vi "SwapElectrodes.vi"(1 "index 2":i32=5, 2 "index 1":i32=4, 3 "Excitations in":dbl[](array[numeric])=[-7.852284145732824, -6.6524880255455034, -6.63672624222675, -6.6562009105673745, -7.978464811675144, -7.977669192926473, -7.983560531970807, -0.0001659795114891018, 0.0, 0.0, 0.0, 0.0, 0.0, 0.0, 0.0, 0.6666666666666666]) -> (0 "Excitations out":dbl[](array[numeric])=[-7.852284145732824, -6.6524880255455034, -6.63672624222675, -6.6562009105673745, -7.977669192926473, -7.978464811675144, -7.983560531970807, -0.0001659795114891018, 0.0, 0.0, 0.0, 0.0, 0.0, 0.0, 0.0, 0.6666666666666666])   [LabVIEW 2018]
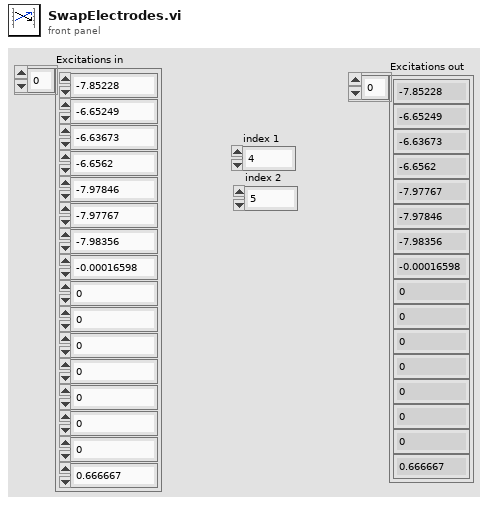
[diagram p1: front panel]
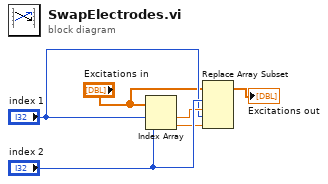
[diagram p0: block diagram]
diagram:
  n1 = Index Array(array="Excitations in", index #1="index 1", index #2="index 2") -> (element #1=w5:dbl, element #2=w4:dbl)
  n2 = Replace Array Subset(array="Excitations in", new element #1=w5, index #1="index 2", new element #2=w4, index #2="index 1") -> (→"Excitations out":dbl[])
